vi "ClearDependencies.vi"(8 "error in (no error)":errorcluster, 11 "SMO in":refnum<class "SMO.lvclass">) -> (0 "error out":errorcluster, 3 "SMO out":refnum<class "SMO.lvclass">)   [LabVIEW 2021, in "smo.lvlib" / "SMO.lvclass"]
uses:
  SMO.lvclass
  Support/Attribute.Dependencies/Attribute.Dependencies.lvclass
  C:/Repositories/SMO/src/Support/Attribute/Attribute.lvclass
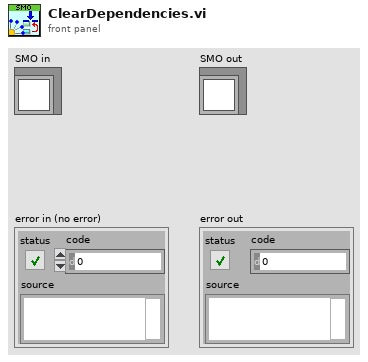
[diagram p1: front panel]
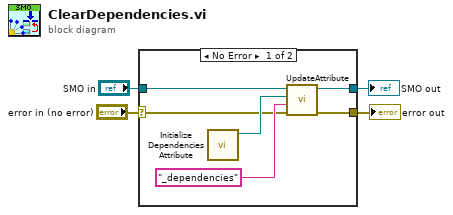
[diagram p0: block diagram]
diagram:
  n1 = case shown="No Error" "error in (no error)" {
    selector: "error in (no error)" -> [w5 w11]
    tunnel: "SMO in" -> [w8 w12]
    tunnel: [w7 w11] -> w3
    tunnel: [w6 w12] -> w2
    frame No Error {
      n2 = call "Initialize Dependencies Attribute.vi"() -> ("Attribute.Dependencies"=w9:refnum<class "Attribute.Dependencies.lvclass">)  [unwired: 11 in]
      n3 = call "UpdateAttribute.vi"("error in (no error)"=w5, "Attribute Name"="_dependencies" ("name"), "Attribute"=w9, "SMO in"=w8) -> ("error out"=w7:errorcluster, "SMO out"=w6:refnum<class "SMO.lvclass">)  [unwired: 5 in, 1 out]
    }
    frame Error {
    }
  }
  "SMO out" <- w2
  "error out" <- w3
